vi "Unbundle and Filter MCL Rows.vi"(7 "filter changed items":bool, 8 "error in":errorcluster, 11 "refresh items":T2[](array[typedef])) -> (0 "error out":errorcluster, 1 "background colors":u32[][](array[colorbox]), 2 "item symbols":T1[](array[typedef])=[enum."Blank", enum."Port", enum."Remote Terminal", enum."Subaddress", enum."Bus Controller", enum."Parameter"], 3 "item names":string[][](array[string]))   [LabVIEW 2020, in "AIM MIL-STD-1553 System Explorer.lvlib" / "Implementation.lvlib" / "Refresh.lvlib"]
uses:
  Refresh.lvlib
  Change Type.ctl
  MCL Row.ctl
  Symbols.ctl
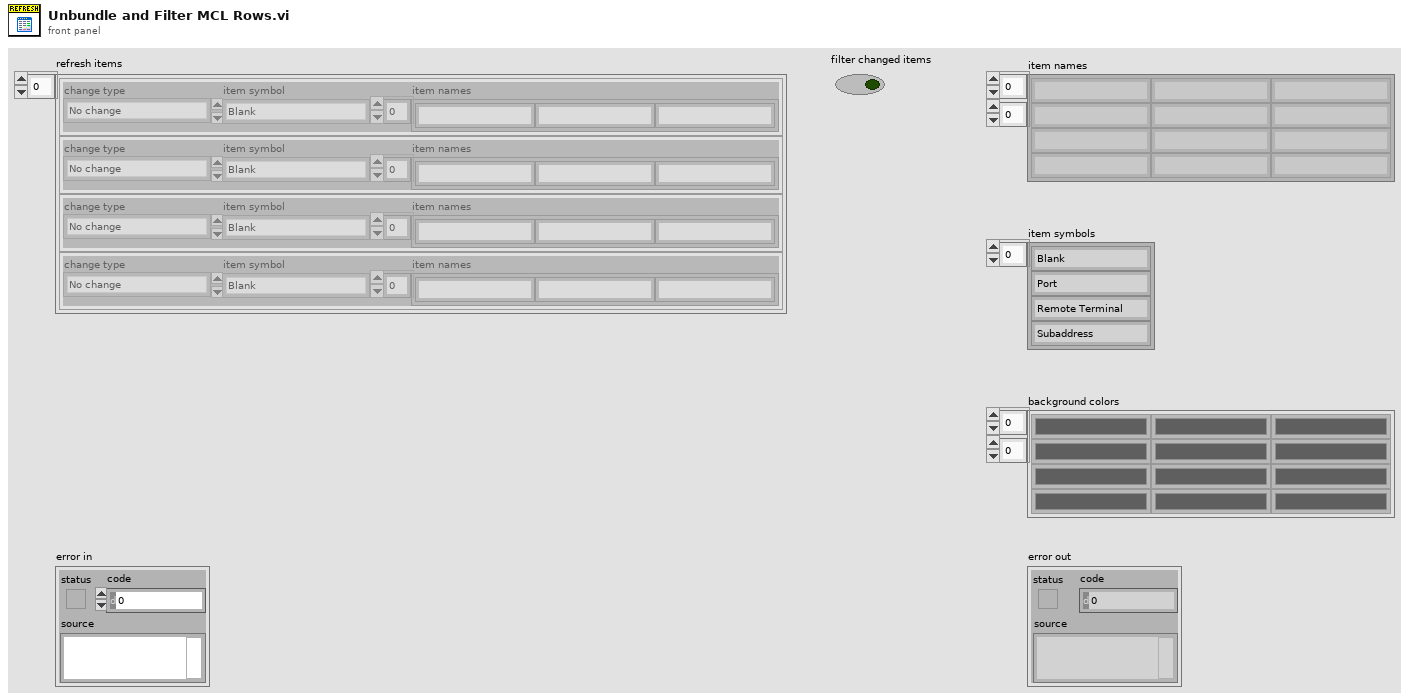
[diagram p1: front panel]
types:
  T1 = typedef "AIM MIL-STD-1553 System Explorer.lvlib/Implementation.lvlib/Refresh.lvlib/Symbols.ctl" = enum16{"Blank", "MIL-STD-1553", "Port", "Remote Terminal", "Subaddress", "Bus Controller", "Acyclic Frame", "Mode Code", "Message", "Parameter", "Item"}
  T2 = typedef "AIM MIL-STD-1553 System Explorer.lvlib/Implementation.lvlib/Refresh.lvlib/MCL Row.ctl" = cluster{"change type":T3, "item symbol":T1, "item names":string[]}
  T3 = typedef "AIM MIL-STD-1553 System Explorer.lvlib/Implementation.lvlib/Refresh.lvlib/Change Type.ctl" = enum16{"No change", "Modify", "Add", "Remove"}
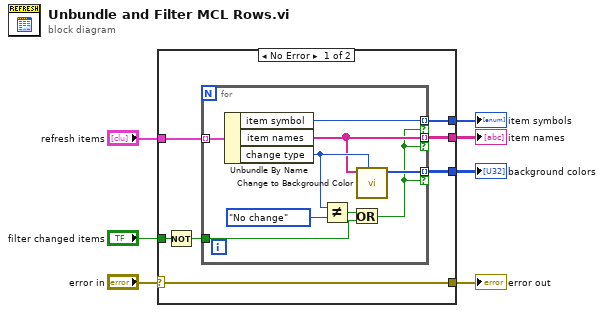
[diagram p0: block diagram]
diagram:
  n1 = case shown="No Error" "error in" {
    selector: "error in" -> [w8 w24]
    tunnel: "refresh items" -> [w14 _]
    tunnel: "filter changed items" -> [w13 _]
    tunnel: [w11 _] -> w5
    tunnel: [w10 _] -> w4
    tunnel: [w9 _] -> w3
    tunnel: [w8 w24] -> w1
    frame No Error {
      n2 = Not(x=w13) -> (.not. x?=w12:bool)
      n3 = for {
        tunnel: w14 -> [w23] mode=indexing
        tunnel: w12 -> [w20]
        tunnel: [w19] -> w11 mode=indexing if=w15
        tunnel: [w17] -> w10 mode=indexing if=w15
        tunnel: [w16] -> w9 mode=indexing if=w15
        n4 = Unbundle By Name(w23) -> ("item symbol"=w19:T1, "item names"=w17:string[], "change type"=w18:T3)
        n5 = Not Equal?(x=w18, y=Change_Type."No change") -> (x != y?=w21:bool)
        n6 = Or(x=w21, y=w20) -> (x .or. y?=w15:bool)
        n7 = call "Change to Background Color.vi"("change type"=w18, "item names"=w17) -> ("background colors"=w16:u32[])  [unwired: 9 in]
      }
    }
    frame Error {
    }
  }
  "error out" <- w1
  "item names" <- w4
  "item symbols" <- w5
  "background colors" <- w3
